vi "test-slew-rate-limiter-exec.vi"() -> ()   [LabVIEW 2019]
uses:
  <vilib>/Rock Robotics/WPI/ThirdParty/JAS_Junk/TrajLib/SlewRateLimiter_New.vi
  <vilib>/Rock Robotics/WPI/ThirdParty/JAS_Junk/TrajLib/SlewRateLimiter_Reset.vi
  <vilib>/Rock Robotics/WPI/ThirdParty/JAS_Junk/TrajLib/SlewRateLimiter_Calculate.vi
  <vilib>/Rock Robotics/WPI/ThirdParty/JAS_Junk/TrajLib/SlewRateLimiter_SetRate.vi
  <vilib>/Rock Robotics/WPI/ThirdParty/JAS_Junk/TrajLib/Util_GetTime.vi
  <vilib>/Rock Robotics/WPI/ThirdParty/JAS_Junk/TrajLib/Util_LibraryGlobals.vi
  <vilib>/Rock Robotics/WPI/ThirdParty/JAS_Junk/TrajLib/Trajectory_Library.lvlib
panel:
  out "LibUsage_ProfiledPID":i32 format="%20.0f"
  out "LibUsage_PIDController":i32 format="%20.0f"
  out "LibUsage_Odometry":i32 format="%20.0f"
  out "LibUsage_LinearFIlter":i32 format="%20.0f"
  out "LibUsage_TrapezoidProfile":i32 format="%20.0f"
  out "LibUsage_Kinematics":i32 format="%20.0f"
  in  "Enable":bool=TRUE
  in  "Rate Limit":dbl=9999.0
  out "Waveform Chart":cluster{dbl, dbl}(graph)
  in  "Frequency":dbl(slide)=0.2 min=0.1 max=1000.0 step=0.5 scale=0.1..10.0
  in  "Amplitude":dbl(slide)=1.0 scale=0.0..10.0
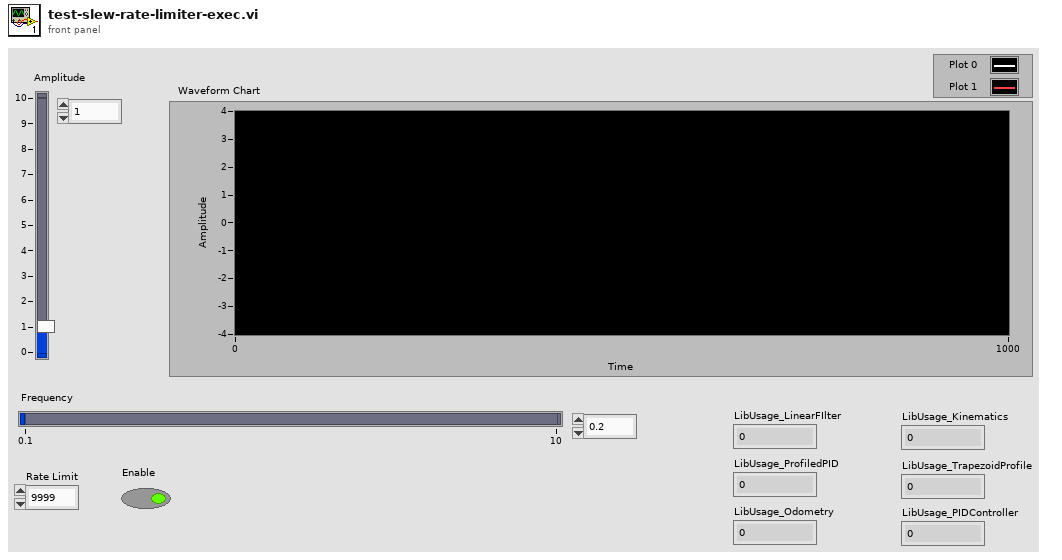
[diagram p1: front panel]
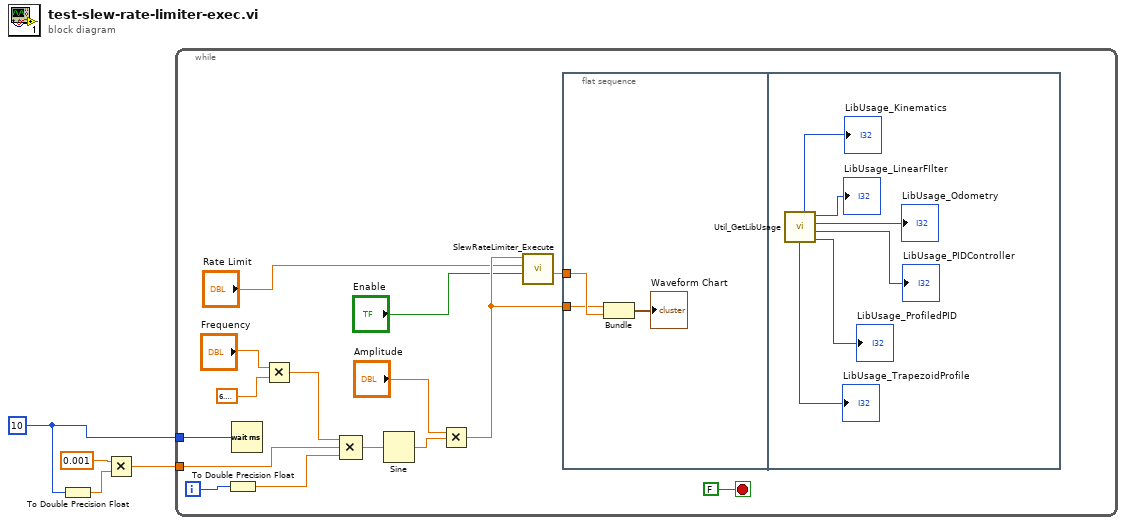
[diagram p0: block diagram]
diagram:
  w2 = u32 10 ("milliseconds to wait")
  n1 = To Double Precision Float(number=w2) -> (double precision float=w3:dbl)
  n2 = Multiply(x=0.001 ("value"), y=w3) -> (x*y=w1:dbl)
  n3 = while {
    tunnel: w2 -> [w11]
    tunnel: w1 -> [w9]
    i -> [w18]
    stop <- FALSE stop-if-true
    n4 = To Double Precision Float(number=w18) -> (double precision float=w17:dbl)
    n5 = Wait (ms)(milliseconds to wait=w11) -> ()  [unwired: 1 out]
    n6 = Multiply(x="Frequency", y=6.283185307179586) -> (x*y=w10:dbl)
    n7 = Compound Arithmetic op=MULTIPLY(w10, w9, w17) -> (w16:dbl)
    n8 = Sine(x=w16) -> (sin(x)=w15:dbl)
    n9 = Multiply(x="Amplitude", y=w15) -> (x*y=w7:dbl)
    n10 = call <vilib>:"SlewRateLimiter_Execute.vi"("Enable"="Enable", "Rate"="Rate Limit", "Input"=w7) -> ("Output"=w8:dbl)  [unwired: 7 in, 1 out]
    n11 = flat-sequence {
      tunnel: w8 -> [w21]
      tunnel: w7 -> [w20]
      frame #0 {
        n12 = Bundle(w20, "Output"=w21) -> (→"Waveform Chart":cluster{dbl, "Output":dbl})  [unwired: 1 in]
      }
      frame #1 {
        n13 = call <vilib>:"Util_GetLibUsage.vi"() -> ("LibUsage_ProfiledPID"=→"LibUsage_ProfiledPID":i32, "LibUsage_PIDController"=→"LibUsage_PIDController":i32, "LibUsage_Odometry"=→"LibUsage_Odometry":i32, "LibUsage_LinearFIlter"=→"LibUsage_LinearFIlter":i32, "LibUsage_TrapezoidProfile"=→"LibUsage_TrapezoidProfile":i32, "LibUsage_Kinematics"=→"LibUsage_Kinematics":i32)  [unwired: 6 in]
      }
    }
  }
